vi "test Create Empty File.vi"(8 "error in (no error)":errorcluster, 11 "TestCase in":refnum<class "Configuration Tests.lvclass">) -> (0 "error out":errorcluster, 3 "TestCase out":refnum<class "Configuration Tests.lvclass">)   [LabVIEW 2017, in "Configuration Tests.lvclass"]
uses:
  Configuration Tests.lvclass
  Typedefs/DSF Version Info.ctl
  <vilib>/addons/_JKI Toolkits/VI Tester/TestCase.llb/TestCase.lvclass
  Classes/Configuration/Configuration Session.lvclass
  DSF Core.lvlib
  C:/Program Files (x86)/National Instruments/LabVIEW 2017/vi.lib/addons/_JKI Toolkits/VI Tester/TestCase.llb/TestCase.lvclass
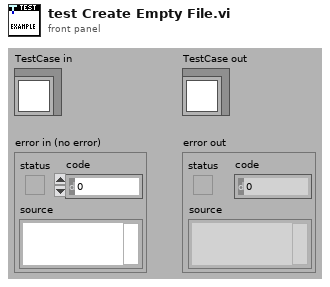
[diagram p1: front panel]
types:
  T1 = typedef "DSF Core.lvlib/DSF Version Info.ctl" = cluster{"major":u32, "minor":u32, "fix":u32, "build":string}
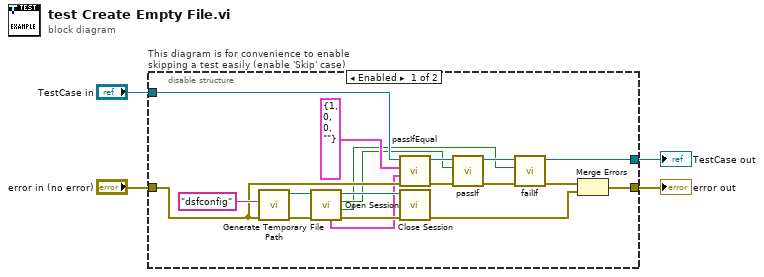
[diagram p0: block diagram]
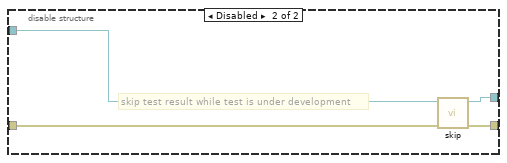
[diagram p2: hidden frame]
diagram:
  n1 = disable-structure "This diagram is for convenience to enable skipping a test easily (enable 'Skip' case)" shown="Enabled" {
    disable-tunnel: "TestCase in" -> [w20 w27]
    disable-tunnel: [w6 w25] -> w1
    disable-tunnel: [w18 w26] -> w3
    disable-tunnel: "error in (no error)" -> [w19 w24]
    frame Enabled {
      n2 = call <vilib>:"Generate Temporary File Path.vi"("error in (no error)"=w19, "Temporary File Extension (tmp)"="dsfconfig") -> ("error out"=w22:errorcluster, "Unique Temporary File Path"=w23:path)  [unwired: 8 in]
      n3 = call "Open Session.vi"("error in (no error)"=w22, "configuration file path"=w23) -> ("error out"=w16:errorcluster, "file replaced?"=w5:bool, "file created?"=w9:bool, "configuration session"=w15:refnum<class "Configuration Session.lvclass">, "version"=w13:T1)  [unwired: 5 in]
      n4 = call-dynamic "passIfEqual.vi"("error in (no error)"=w19, "y"=w13, "x"=T1 {"major"=1, "minor"=0, "fix"=0, "build"=""} ("version"), "TestCase in"=w20) -> ("error out"=w17:errorcluster, "TestCase out"=w10:refnum<class "Configuration Tests.lvclass">)  [unwired: 6 in]
      n5 = call "Close Session.vi"("error in (no error)"=w16, "configuration session"=w15) -> ("error out"=w14:errorcluster)  [unwired: 8 in, 1 out]
      n6 = call-dynamic "passIf.vi"("error in (no error)"=w17, "pass"=w9, "TestCase in"=w10) -> ("error out"=w11:errorcluster, "TestCase out"=w7:refnum<class "Configuration Tests.lvclass">)  [unwired: 7 in]
      n7 = call-dynamic "failIf.vi"("error in (no error)"=w11, "fail"=w5, "TestCase in"=w7) -> ("error out"=w8:errorcluster, "TestCase out"=w6:refnum<class "Configuration Tests.lvclass">)  [unwired: 7 in]
      n8 = Merge Errors(w8, w14) -> (w18:errorcluster)
    }
    frame Disabled {
      # "skip test result while test is under development"
      n9 = call <vilib>:"skip.vi"("error in (no error)"=w24, "TestCase in"=w27) -> ("error out"=w26:errorcluster, "TestCase out"=w25:refnum<class "Configuration Tests.lvclass">)  [unwired: 8 in]
    }
  }
  "error out" <- w3
  "TestCase out" <- w1
